vi "Serialize.vi"(8 "error in":errorcluster, 9 "OwningElement in":refnum<k20>, 10 "Document in":refnum<k20>, 11 "RealMeasure in":refnum<class "RealMeasure.lvclass">) -> (0 "error out":errorcluster, 1 "OwningElement out":refnum<k20>, 2 "Document out":refnum<k20>, 3 "RealMeasure out":refnum<class "RealMeasure.lvclass">)   [LabVIEW 2021, in "ProligentXMLGenerator.lvlib" / "RealMeasure.lvclass"]
uses:
  RealMeasure.lvclass
  RealMeasure.lvclass/RealMeasure.ctl
  Base/DOMSupport/DOMSupport.lvlib
  Measure/Measure.lvclass
  <vilib>/xml/NI_XML.lvlib
  <vilib>/xml/Close Reference(Node).vi
  MeasureLimit/MeasureLimit.lvclass
  Base/Decimal/Decimal.lvclass
  C:/Projects/proligent-xml-generator-labview/src/ProligentXMLGenerator/Measure/Measure/Measure.lvclass
  Base/UnsignedByte/UnsignedByte.lvclass
  C:/Projects/proligent-xml-generator-labview/src/ProligentXMLGenerator/Base/Attribute/Attribute.lvclass
  C:/Projects/proligent-xml-generator-labview/src/ProligentXMLGenerator/Base/UnsignedByte/UnsignedByte.lvclass
  Base/MeasureKind/MeasureKind.lvclass
  C:/Projects/proligent-xml-generator-labview/src/ProligentXMLGenerator/Base/MeasureKind/MeasureKind.lvclass
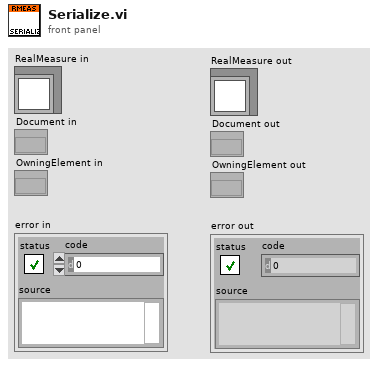
[diagram p1: front panel]
types:
  T1 = typedef "ProligentXMLGenerator.lvlib/RealMeasure.lvclass/Data.ctl" = cluster{"Value":refnum<class "Decimal.lvclass">, "Precision":refnum<class "UnsignedByte.lvclass">}
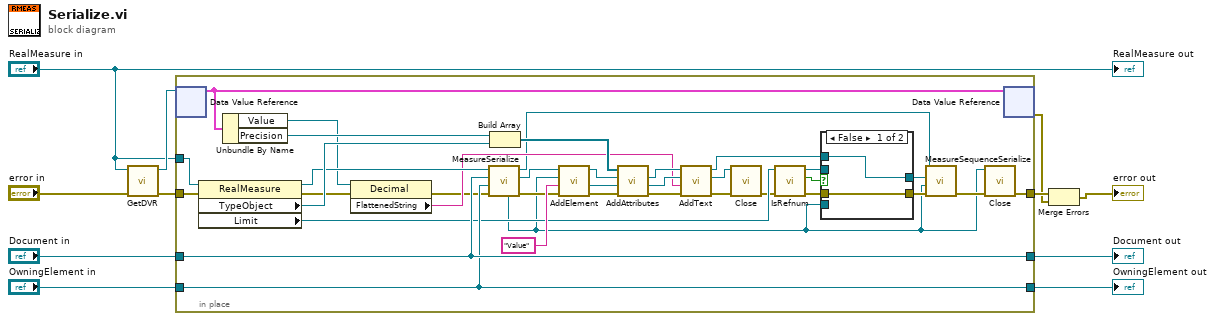
[diagram p0: block diagram]
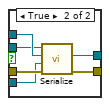
[diagram p2: hidden frame]
diagram:
  n1 = call "GetDVR.vi"("error in"="error in", "RealMeasure"="RealMeasure in") -> ("error out"=w4:errorcluster, "DVRReference"=w3:refnum<data-value>)  [unwired: 8 in]
  n2 = in-place "In Place Element Structure" {
    in-place-border: [w38] -> w5
    in-place-border: "Document in" -> [w45]
    in-place-border: w4 -> [w44]
    in-place-border: "OwningElement in" -> [w43]
    in-place-border: [w43] -> w7
    in-place-border: [w45] -> w6
    in-place-border: "RealMeasure in" -> [w41]
    n3 = in-place-dvr #1(w3) -> (w47:T1)  [unwired: 1 out]
    n4 = property on="Property Node" class="RealMeasure"(reference=w41, error in=w44) -> (reference out=w32:refnum<class "RealMeasure.lvclass">, error out=w17:errorcluster, "TypeObject"=w33:refnum<class "MeasureKind.lvclass">, "Limit"=w25:refnum<class "MeasureLimit.lvclass">)
    n5 = Unbundle By Name(w47) -> ("Value"=w19:refnum<class "Decimal.lvclass">, "Precision"=w31:refnum<class "UnsignedByte.lvclass">)
    n6 = property on="Property Node" class="Decimal"(reference=w19, error in=w17) -> (error out=w16:errorcluster, "FlattenedString"=w18:string)  [unwired: 1 out]
    n7 = call "MeasureSerialize.vi"("error in"=w16, "OwningElement in"=w43, "Document in"=w45, "Measure in"=w32) -> ("error out"=w29:errorcluster, "Document out"=w30:refnum<k20>, "Measure in"=w14:refnum<class "RealMeasure.lvclass">, "Element"=w12:refnum<k20>)  [unwired: 3 in, 1 out]
    n8 = Build Array(w31, w33) -> (w46:refnum<class "Attribute.lvclass">[])
    n9 = call "AddElement.vi"("error in"=w29, "Name"="Value", "OwningElement in"=w12, "Document in"=w30) -> ("error out"=w37:errorcluster, "NewElement"=w39:refnum<k20>, "Document out"=w40:refnum<k20>)  [unwired: 4 in, 1 out]
    n10 = call "AddAttributes.vi"("error in"=w37, "OwningElement in"=w39, "Document in"=w40, "Attributes"=w46) -> ("error out"=w36:errorcluster, "OwningElement out"=w34:refnum<k20>, "Document out"=w35:refnum<k20>)  [unwired: 5 in]
    n11 = call "AddText.vi"("error in"=w36, "Text"=w18, "OwningElement in"=w34, "Document in"=w35) -> ("error out"=w21:errorcluster, "OwningElement out"=w22:refnum<k20>, "Document out"=w24:refnum<k20>)  [unwired: 5 in]
    n12 = call-poly <vilib>:"Close.vi"("error in (no error)"=w21, "node"=w22) -> ("error out"=w20:errorcluster)  [unwired: 7 in]
    n13 = call "IsRefnum.vi"("error in"=w20, "MeasureLimit in"=w25) -> ("error out"=w28:errorcluster, "IsRefnum"=w27:bool, "MeasureLimit out"=w26:refnum<class "MeasureLimit.lvclass">)  [unwired: 7 in]
    n14 = case shown="False" w27 {
      tunnel: w28 -> [w49 w53]
      tunnel: [w49 w55] -> w23
      tunnel: w26 -> [_ w52]
      tunnel: w24 -> [w48 w54]
      tunnel: w12 -> [_ w51]
      tunnel: [w48 w50] -> w13
      frame False {
      }
      frame True {
        n15 = call "Serialize.vi"("error in"=w53, "OwningElement in"=w51, "Document in"=w54, "MeasureLimit in"=w52) -> ("error out"=w55:errorcluster, "Document out"=w50:refnum<k20>)  [unwired: 4 in, 2 out]
      }
    }
    n16 = call "MeasureSequenceSerialize.vi"("error in"=w23, "OwningElement in"=w12, "Document in"=w13, "Measure in"=w14) -> ("error out"=w15:errorcluster)  [unwired: 4 in, 3 out]
    n17 = call-poly <vilib>:"Close.vi"("error in (no error)"=w15, "node"=w12) -> ("error out"=w38:errorcluster)  [unwired: 7 in]
    n18 = in-place-dvr #1(w47) -> (w2:errorcluster)  [unwired: 1 out]
  }
  "Document out" <- w6
  "OwningElement out" <- w7
  n19 = Merge Errors(w5, w2) -> (→"error out":errorcluster)
  "RealMeasure out" <- "RealMeasure in"
